vi "IsItemParent.vi"(8 "error in (no error)":errorcluster, 9 "Item to compare":refnum<class "ILabVIEWItem.lvclass">, 11 "CLabVIEWItem in":refnum<class "CLabVIEWItem.lvclass">) -> (0 "error out":errorcluster, 2 "Is parent?":bool, 3 "CLabVIEWItem out":refnum<class "CLabVIEWItem.lvclass">)   [LabVIEW 2020, in "LabVIEWItem.lvlib" / "CLabVIEWItem.lvclass"]
uses:
  CLabVIEWItem.lvclass
  LabVIEWObjectInterfaces/ILabVIEWItem/ILabVIEWItem.lvclass
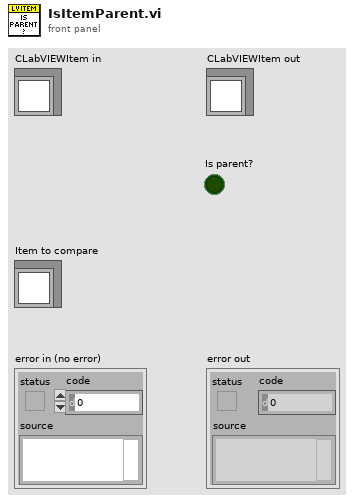
[diagram p1: front panel]
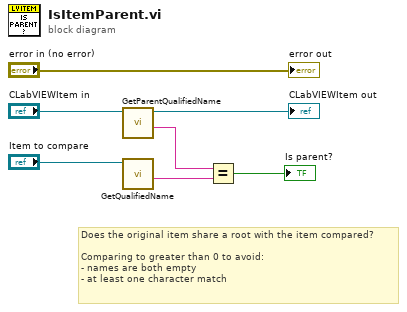
[diagram p0: block diagram]
diagram:
  # "Does the original item share a root with the item compared?\n\nComparing to greater than 0 to avoid:\n- names are both empty\n- at least one character match"
  n1 = call-dynamic "GetParentQualifiedName.vi"("CLabVIEWItem in"="CLabVIEWItem in") -> ("Name"=w3:string, "CLabVIEWItem out"=→"CLabVIEWItem out":refnum<class "CLabVIEWItem.lvclass">)  [unwired: 8 in, 1 out]
  n2 = call-dynamic "GetQualifiedName.vi"("ILabVIEWItem in"="Item to compare") -> ("Qualified name"=w2:string)  [unwired: 8 in, 2 out]
  n3 = Equal?(x=w3, y=w2) -> (x = y?=→"Is parent?":bool)
  "error out" <- "error in (no error)"
